vi "xijk_load_from_file_is_cube_file.vi"(7 "filepaths in":T1, 8 "error in":errorcluster, 11 "file path in":path) -> (0 "error out":errorcluster, 5 "filepaths out":T1)   [LabVIEW 2010]
uses:
  Type Def/filepath.ctl
  xijk_combined_file.lvlib
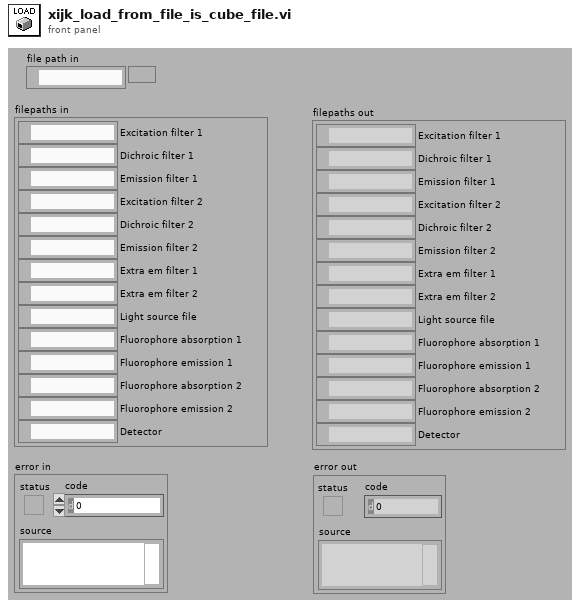
[diagram p1: front panel]
types:
  T1 = typedef "filepath.ctl" = cluster{"Excitation filter 1":path, "Dichroic filter 1":path, "Emission filter 1":path, "Excitation filter 2":path, "Dichroic filter 2":path, "Emission filter 2":path, "Extra em filter 1":path, "Extra em filter 2":path, "Light source file":path, "Fluorophore absorption 1":path, "Fluorophore emission 1":path, "Fluorophore absorption 2":path, "Fluorophore emission 2":path, "Detector":path}
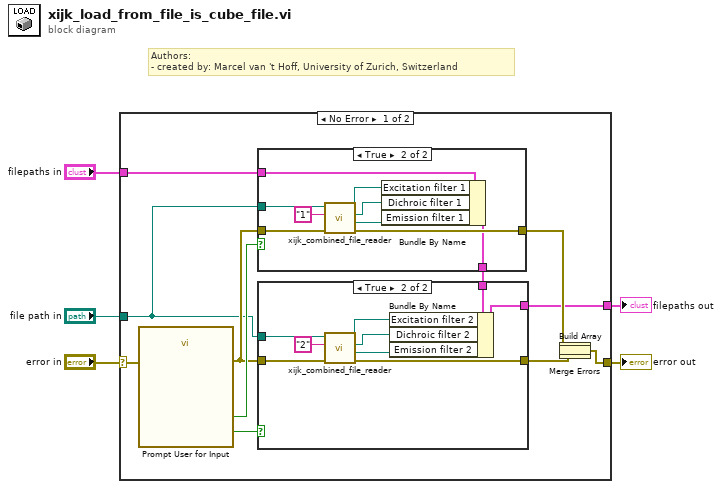
[diagram p0: block diagram]
diagram:
  # "Authors: \n- created by: Marcel van 't Hoff, University of Zurich, Switzerland"
  n1 = case shown="No Error" "error in" {
    selector: "error in" -> [w15 w41]
    tunnel: [w11 w41] -> w5
    tunnel: "file path in" -> [w10 _]
    tunnel: "filepaths in" -> [w9 w40]
    tunnel: [w7 w40] -> w1
    frame No Error {
      n2 = call "Prompt User for Input"("error in (no error)"=w15) -> ("Channel 2"=w16:bool, "Channel 1"=w17:bool, "error out"=w14:errorcluster)  [unwired: 15 in, 1 out]
      n3 = case shown="True" w17 {
        tunnel: w10 -> [_ w37]
        tunnel: w14 -> [w30 w39]
        tunnel: [w30 w38] -> w13
        tunnel: w9 -> [w29 w35]
        tunnel: [w29 w34] -> w8
        frame False {
        }
        frame True {
          n4 = call "xijk_combined_file_reader.vi"("error in"=w39, "channel"="1", "file path input"=w37) -> ("error out"=w38:errorcluster, "file path out EM"=w31:path, "file path out BS"=w32:path, "file path out EX"=w33:path)  [unwired: 5 in]
          n5 = Bundle By Name(cluster=w35, "Excitation filter 1"=w33, "Dichroic filter 1"=w32, "Emission filter 1"=w31) -> (w34:T1)
        }
      }
      n6 = case shown="True" w16 {
        tunnel: w10 -> [_ w26]
        tunnel: w14 -> [w19 w28]
        tunnel: [w19 w27] -> w12
        tunnel: w8 -> [w18 w24]
        tunnel: [w18 w20] -> w7
        frame False {
        }
        frame True {
          n7 = call "xijk_combined_file_reader.vi"("error in"=w28, "channel"="2", "file path input"=w26) -> ("error out"=w27:errorcluster, "file path out EM"=w21:path, "file path out BS"=w22:path, "file path out EX"=w23:path)  [unwired: 5 in]
          n8 = Bundle By Name(cluster=w24, "Excitation filter 2"=w23, "Dichroic filter 2"=w22, "Emission filter 2"=w21) -> (w20:T1)
        }
      }
      n9 = Build Array(w13, w12) -> (w6:errorcluster[])
      n10 = Merge Errors(w6) -> (w11:errorcluster)
    }
    frame Error {
    }
  }
  "error out" <- w5
  "filepaths out" <- w1
